vi "Log_data_tab_ligne.vi"(7 "in":refnum<file>, 8 "errin":errorcluster, 9 "Tableau":T2(array[cluster]), 10 "test number":string="OCVACIR : ", 11 "test name":string="OCVACIR : ") -> (0 "sortie d'erreur":errorcluster caption="errout", 5 "refnum en sortie":refnum<file>)   [LabVIEW 2020]
doc: "Ajoute une ligne de log dans le fichier"
uses:
  <userlib>/Alex Log/Log_ligne.ctl
panel:
  in  "date?":bool=TRUE
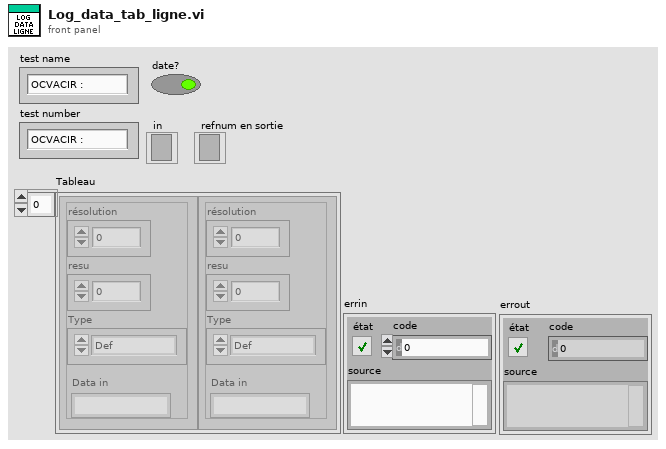
[diagram p1: front panel]
types:
  T1 = typedef "Log_ligne.ctl" = enum16{"Def", "Volt V", "Volt mV", "ohm Ohm", "ohm mOhm", "ohm kOhm", "ohm MOhm", "Opérateur", "EPI", "SN"}
  T2 = cluster{"résolution":i16, "resu":dbl, "Type":T1, "Data in":string}[]
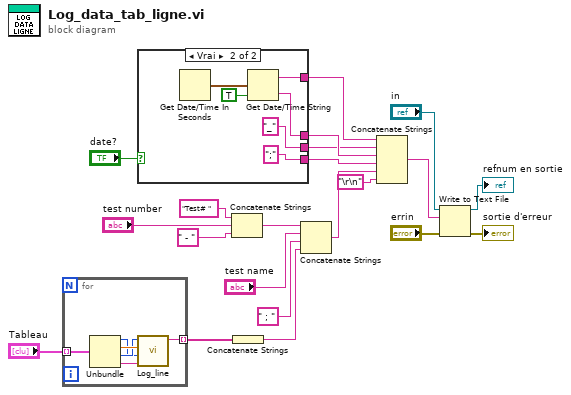
[diagram p0: block diagram]
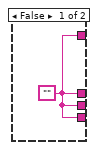
[diagram p2: hidden frame]
diagram:
  n1 = for {
    tunnel: "Tableau" -> [w27] mode=indexing
    tunnel: [w23] -> w16 mode=indexing
    n2 = Unbundle(w27) -> ("résolution"=w24:i16, "resu"=w26:dbl, "Type"=w25:T1, "Data in"=w22:string)
    n3 = call <userlib>:"Log_line.vi"("Data str"=w22, "résolution"=w24, "resu"=w26, "Type"=w25) -> ("message"=w23:string)  [unwired: 7 in]
  }
  n4 = case shown="Vrai" "date?" {
    tunnel: [w28 w34] -> w10
    tunnel: [w28 w33] -> w9
    tunnel: [w28 "_" ("chaîne")] -> w5
    tunnel: [w28 ";" ("chaîne")] -> w2
    frame False {
      w28 = ""
    }
    frame True {
      n5 = Get Date/Time In Seconds() -> (seconds since 1Jan1904=w32:timestamp)
      n6 = Get Date/Time String(seconds (now)=w32, want seconds? (F)=TRUE ("secondes ? (F)")) -> (date string=w33:string, time string=w34:string)  [unwired: 1 in]
    }
  }
  n7 = Concatenate Strings("Test# " ("chaîne"), "test number", " - " ("chaîne")) -> (w17:string)
  n8 = Concatenate Strings(w16) -> (w15:string)
  n9 = Concatenate Strings(w17, "test name", " ; " ("chaîne"), w15) -> (w1:string)
  n10 = Concatenate Strings(w9, w5, w10, w2, w1, "\r\n") -> (w6:string)
  n11 = Write to Text File(file (use dialog)="in", text=w6, error in="errin") -> (refnum out=→"refnum en sortie":refnum<file>, error out=→"sortie d'erreur":errorcluster)  [unwired: 1 in, 1 out]
